vi "GOMDBTS2048 spectral Get Lambdas.vi"(8 "error in (no error)":errorcluster, 10 "wavelengthRaster":bool, 11 "handle":i32) -> (0 "error out":errorcluster, 2 "function return":i32, 3 "lambdas":dbl[](array[numeric]))   [LabVIEW 2015, in "GOMDBTS2048.lvlib"]
doc: "GOBTS2048DLL int __stdcall GOMDBTS2048_spectralGetLambdas(int handle, bool wavelengthRaster, double* lambdas);"
uses:
  GOMDBTS2048.lvlib
  runtime/GOMDBTS2048.dll
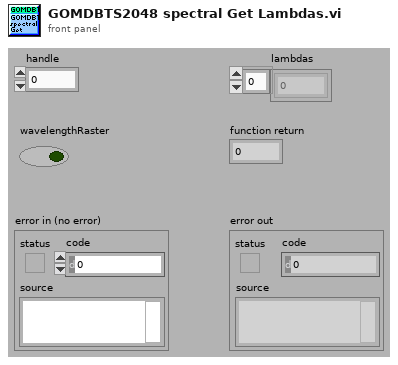
[diagram p1: front panel]
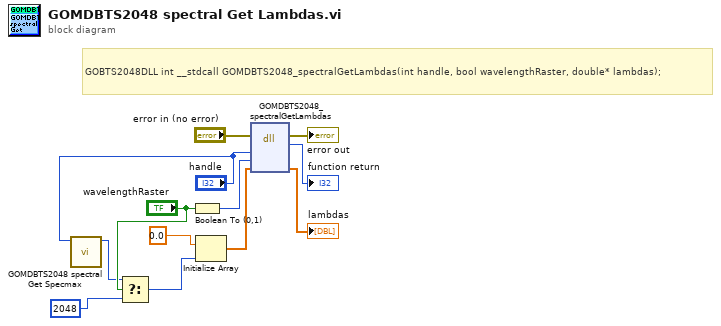
[diagram p0: block diagram]
diagram:
  # "GOBTS2048DLL int __stdcall GOMDBTS2048_spectralGetLambdas(int handle, bool wavelengthRaster, double* lambdas);"
  n1 = call "GOMDBTS2048 spectral Get Specmax.vi"("handle"="handle") -> ("value"=w1:i32)  [unwired: 8 in, 2 out]
  n2 = Select(t=w1, s="wavelengthRaster", f=2048 ("dimension size")) -> (s? t:f=w3:i32)
  n3 = Boolean To (0,1)(Boolean="wavelengthRaster") -> (0, 1=w11:i16)
  n4 = Initialize Array(0.0 ("element"), w3) -> (w10:dbl[])
  n5 = dll-call lib="C:/Users/rkoch/Documents/GO_Library/runtime/GOMDBTS2048.*" fn="GOMDBTS2048_spectralGetLambdas"(error in="error in (no error)", "handle"="handle", "wavelengthRaster"=w11, "lambdas"=w10) -> (error out=→"error out":errorcluster, "return type"=→"function return":i32, "lambdas"=→"lambdas":dbl[])  [unwired: 4 in, 1 out]
